vi "ImportParameterFromFile.vi"(2 "error in (no error)":errorcluster, 3 "fileName":string, 4 "axis in":cluster{"keyHandle":u32, "nodeId":u16}={"keyHandle"=0, "nodeId"=1}) -> (0 "error out":errorcluster {"code" format="%.0x"}, 1 "axis out":cluster{"keyHandle":u32, "nodeId":u16}={"keyHandle"=0, "nodeId"=1})   [LabVIEW 2019, in "maxonEPOS.lvlib"]
doc: "<B>ImportParameterFromFile</B> writes parameters from a file to the device. No message box will be shown."
uses:
  Examples/maxonEPOS.lvlib
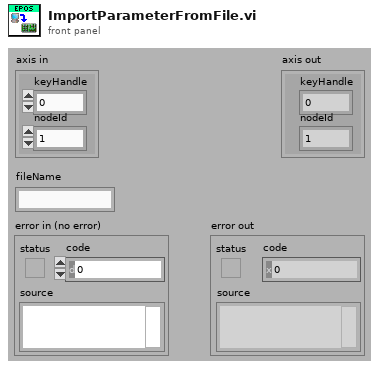
[diagram p1: front panel]
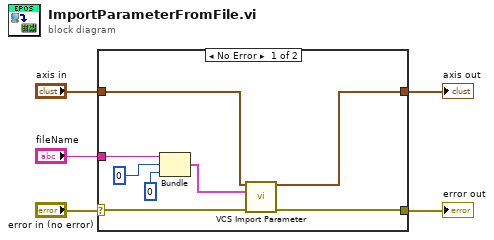
[diagram p0: block diagram]
diagram:
  n1 = case shown="No Error" "error in (no error)" {
    selector: "error in (no error)" -> [w9 w15]
    tunnel: [w8 w15] -> w4
    tunnel: "fileName" -> [w13 _]
    tunnel: [w7 w14] -> w2
    tunnel: "axis in" -> [w6 w14]
    frame No Error {
      n2 = Bundle("fileName"=w13, 0, 0) -> (w10:cluster{"fileName":string, i32, i32})  [unwired: 1 in]
      n3 = call "VCS Import Parameter.vi"("axis in"=w6, "import"=w10, "error in (no error)"=w9) -> ("axis out"=w7:cluster{"keyHandle":u32, "nodeId":u16}, "error out"=w8:errorcluster)  [unwired: 11 in]
    }
    frame Error {
    }
  }
  "error out" <- w4
  "axis out" <- w2
